vi "Rx_with scope_cal_TX.vi"() -> ()   [LabVIEW 2021]
uses:
  use with scope/states_for scope.ctl
  CTL/device_mode.ctl
  <instrlib>/niScope/Controls/niScope trigger source digital.ctl
  use with scope/scope trig type.ctl
  CTL/user config.ctl
  <vilib>/userdefined/High Color/nirio_resource_hc.ctl
  classes/5785_3.2GHz_one channel/5785_3.2GHz_one channel.lvclass
  C:/Users/PXIe8108_Demo/Documents/CHAIM DATA/chaim/5785_sync_for_elbit/tx_pulse/pulse Tx Folder_lv_21/EMEA_ADG_EW_Multi_Emitter_Scenarios/classes/device_type/device_type.lvclass
  classes/5785_2_x_1600MHz/5785_2_x_1600MHz.lvclass
  <instrlib>/niScope/Configure/Trigger/niScope Configure Trigger Edge.vi
  <instrlib>/niScope/Configure/Trigger/niScope Configure Trigger Digital.vi
  <instrlib>/niScope/Acquire/Fetch/niScope Multi Fetch WDT.vi
  <vilib>/Analysis/1siggen.llb/Ramp Pattern by Delta.vi
  classes/device_type/device_type.lvclass
  <vilib>/Analysis/NI_AALBase.lvlib
panel:
  out "delta distance":cluster{dbl[], dbl[]}[](graph)
  out "delta phase (deg)":cluster{dbl[], dbl[]}[](graph)
  in  "niqiest band":dbl[](array[numeric])=[0.0, 0.0, 0.0, 0.0, 0.0, 0.0, 0.0, 0.0, 0.0, 0.0, 0.0, 0.0, 0.0, 0.0, 0.0, 0.0, 0.0, 0.0]
  in  "clear":bool=TRUE
  out "saturate":bool
  out "delta phase(deg) 2":cluster{dbl[], dbl[]}[](graph)
  out "delta amp (dB) 2":cluster{dbl[], dbl[]}[](graph)
  in  "atenuattion (dB)":dbl format="%#_13g"
  in  "Min. Sample Rate":dbl=1250000000.0 format="%#.3p"
  in  "maximum input frequency":dbl=800000000.0 format="%#_13p"
  in  "input impedance":u32(ring)=2 items=["1 mega ohm"=0, "50 ohms"=2]
  in  "keep data":bool=TRUE
  in  "test mode":bool
  in  "save file":bool=TRUE
  in  "file path":path=path "C:/Users/PXIe8108_Demo/Documents/CHAIM DATA/chaim/5785_sync_for_elbit/tx_pulse/pulse Tx Folder_lv_21/EMEA_ADG_EW_Multi_Emitter_Scenarios/data/scope_cal_file.tdms"
  in  "num of recordes":dbl=18.0 format="%#_13g"
  in  "device type":T1=enum."5785 2*1.6GHz"
  in  "num of devices":dbl=2.0 format="%#_13g"
  in  "gen PDW file":bool
  in  "frequncy comb":cluster{"start":dbl, "end":dbl, "delta":dbl}={"start"=20000000.0, "end"=300000000.0, "delta"=1000000.0} {"delta" format="%#_6p"; "end" format="%#_6p"; "start" format="%#_6p"}
  in  "scope cal file":path=path "C:/Users/PXIe8108_Demo/Documents/CHAIM DATA/chaim/5785_sync_for_elbit/tx_pulse/pulse Tx Folder_lv_21/EMEA_ADG_EW_Multi_Emitter_Scenarios/data/scope_cal_file_5171_1234567.tdms"
  out "spectrum":cluster{"f0":dbl, "df":dbl, "magnitude":dbl[]}[](graph)=[{"f0"=0.0, "df"=10000.0, "magnitude"=array[62500 elements]}, {"f0"=0.0, "df"=10000.0, "magnitude"=array[62500 elements]}, {"f0"=0.0, "df"=10000.0, "magnitude"=array[62500 elements]}, {"f0"=0.0, "df"=10000.0, "magnitude"=array[62500 elements]}]
  in  "reset data":bool
  in  "loop mode":bool=TRUE
  out "state":T2=enum."run mesearment"
  in  "cal":bool
  in  "connection table (skip channel 0)":i32[](array[numeric])=[1, 2, 3, 4, 5, 6]
  out "delta amp (dB)":cluster{dbl[], dbl[]}[](graph)
  in  "Channel Name":string="0,1,2,3"
  in  "Resource Name":refnum<k15>="PXI1Slot6" caption="Resource Name(s)"
  in  "amplitude (dB)":dbl=-30.0 format="%#_13g"
  in  "record duration (s)":dbl=0.0001 format="%#_13p"
  out "scope":waveform(dbl)[](graph)=[{"t0"=timestamp(3784724283.659386 s since 1904-01-01), "dt"=8e-10, "Y"=array[125000 elements]}, {"t0"=timestamp(3784724283.659386 s since 1904-01-01), "dt"=8e-10, "Y"=array[125000 elements]}, {"t0"=timestamp(3784724283.659386 s since 1904-01-01), "dt"=8e-10, "Y"=array[125000 elements]}, {"t0"=timestamp(3784724283.659386 s since 1904-01-01), "dt"=8e-10, "Y"=array[125000 elements]}]
  # "scope delta detection"
  # "RF setup"
  # "HW setup"
  # "Rx Data"
  # "scope mapping:\nchannel 0 => 5785_02 _0 \nchannel 1 => 5785_01 _0 \nchannel 2 => 5785_01 _1 \nchannel 3 => 5785_00 _1"
  # "SW setup"
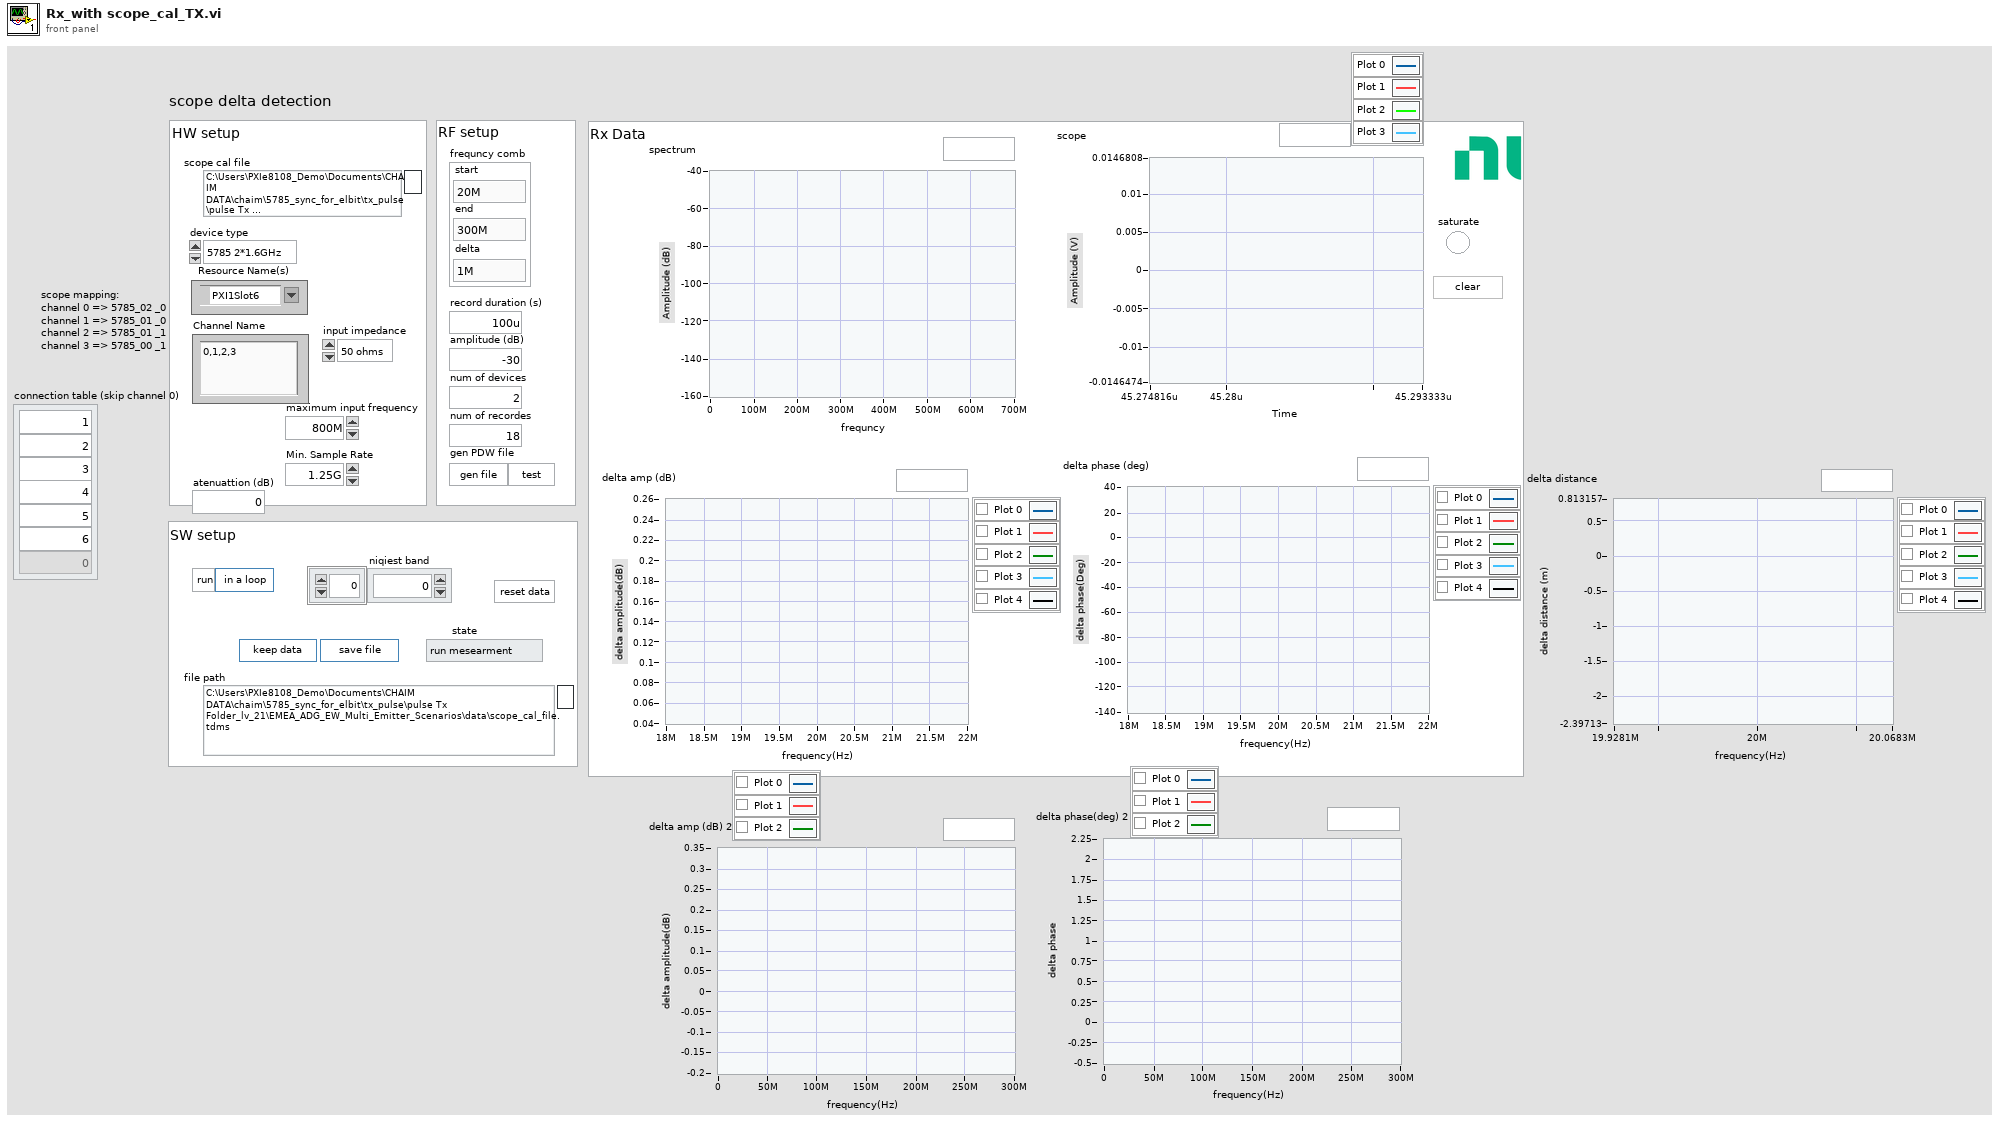
[diagram p1: front panel]
types:
  T1 = typedef "device_mode.ctl" = enum16{"5785 - 3.2GHz", "5785 2*1.6GHz", "P2P - VST", "USRP - 180MHz", "P2P Tx and Rx"}
  T2 = typedef "states_for scope.ctl" = enum16{"wait", "update ME config", "gen secenario", "INI ME", "INI scope", "trig", "close ME", "run mesearment", "save cal data", "get file data", "gen PDW file", "keep the data", "reset memory data", "prime the fifo"}
  T3 = typedef "niScope trigger source digital.ctl" = string
  T4 = typedef "scope trig type.ctl" = enum16{"digital", "analog"}
  T5 = cluster{"freqency":dbl[], "phase":dbl[], "amp":dbl[]}
  T6 = enum16{"open", "open or create", "create or replace", "create", "open (read-only)"}
  T7 = typedef "nirio_resource_hc.ctl" = tag
  T8 = typedef "user config.ctl" = cluster{"vst_device":refnum<k15>[], "RF gain ":dbl, "buffer size":u32, "center frequency (Hz) ":dbl, "P2P sample rate":dbl, "mode":enum16{"USRP - 180MHz", "5785 - 2*180MHz", "5785 - 3.2GHz", "P2P - VST"}, "devicess":T7[], "gen for df":bool, "Rx settings":cluster{"min PW         ":dbl, "max gap        ":dbl, "detection bar":dbl, "peak detect                        ":bool}, "use arb files":bool}
  T9 = cluster{"freqency":dbl[], "phase":dbl[], "amp":dbl[]}[]
  T10 = cluster{"frequncy":dbl, "d amp":dbl, "d phase":dbl}[]
  T11 = cluster{"frequncy":dbl, "d amp":dbl, "d phase":dbl}[][]
  T12 = typedef "PDW_lv2.ctl" = cluster{"t start":dbl, "frequency (Hz)":dbl, "duration (sec)":dbl, "mod type":T13, "mod depth":dbl, "trig":bool, "amp (lin)":dbl, "diraction (deg)":dbl, "phase(deg)":dbl}
  T13 = typedef "mode_type.ctl" = enum8{"CW", "from memory 1", "NC - cw", "LFM", "BPSK", "QPSK"}
  T14 = cluster{"Array":dbl[], "Array":dbl[], "Array":dbl[]}
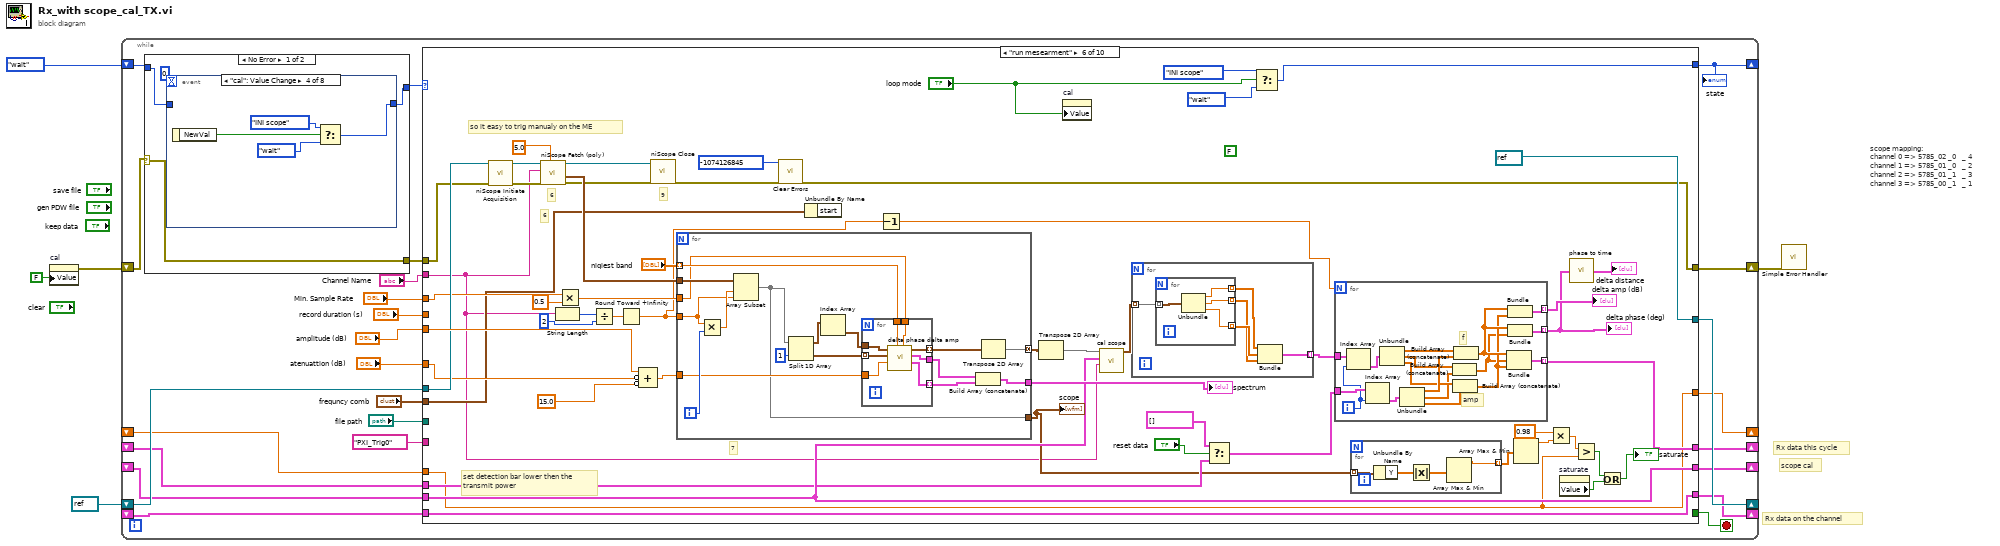
[diagram p0: block diagram]
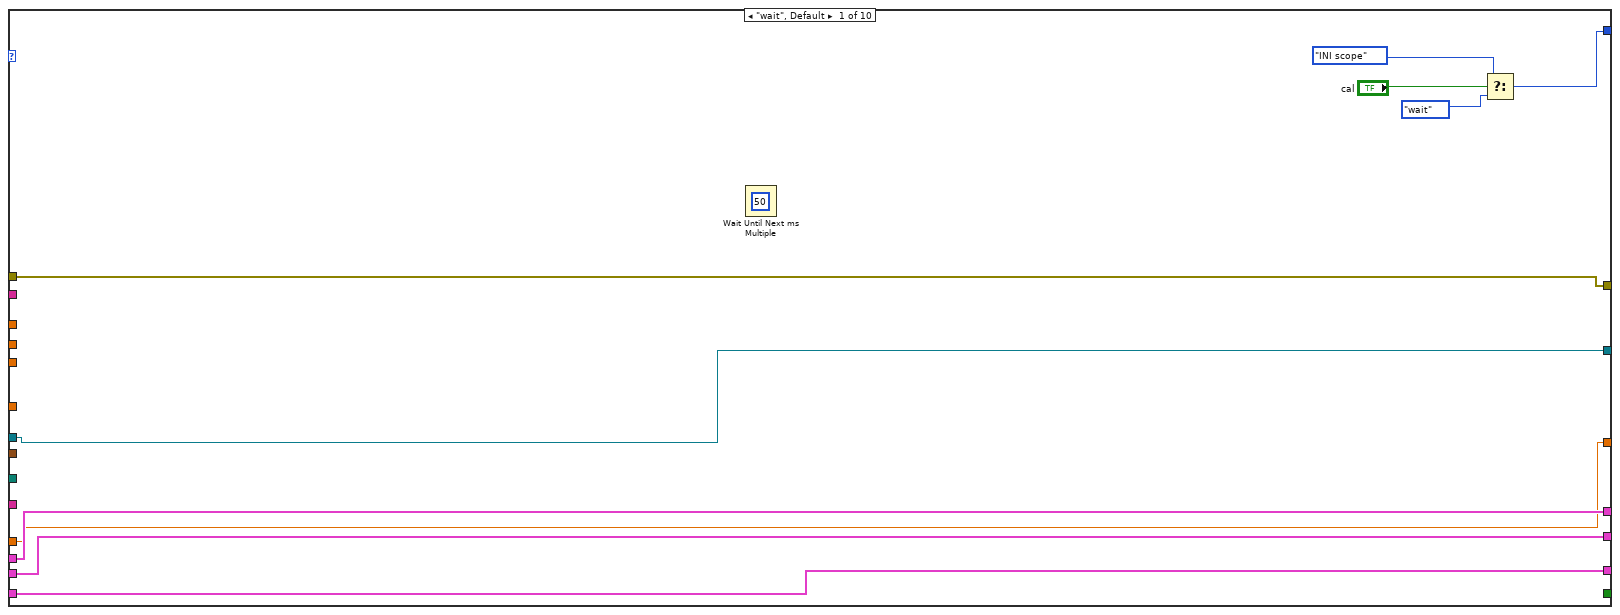
[diagram p2: hidden frame]
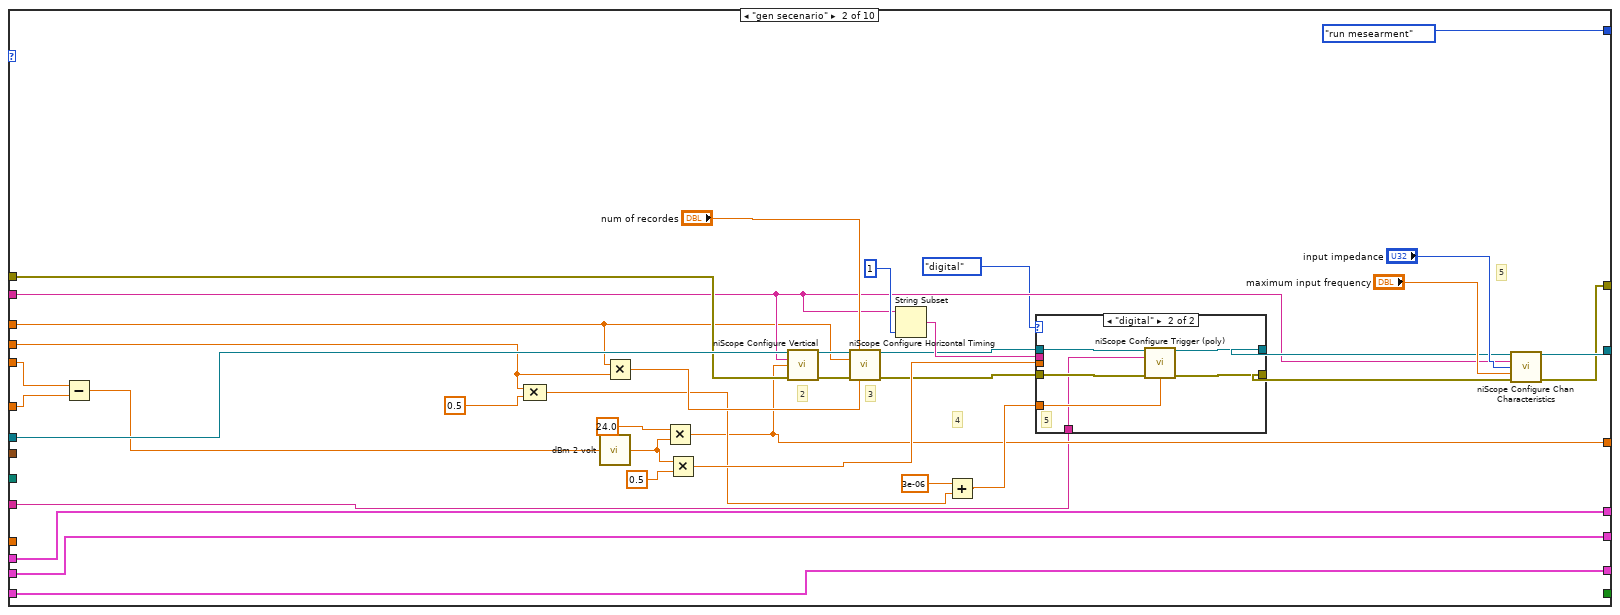
[diagram p3: hidden frame]
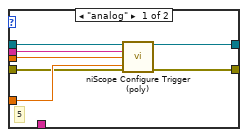
[diagram p4: hidden frame]
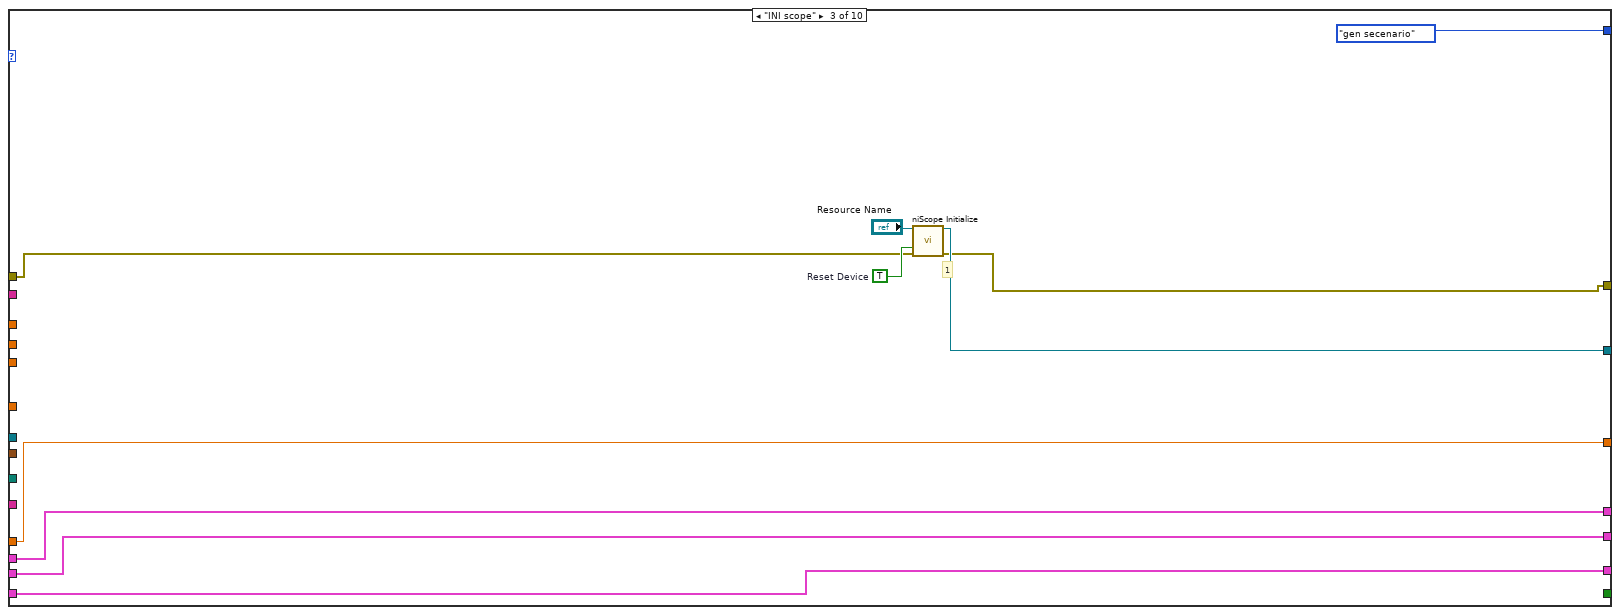
[diagram p5: hidden frame]
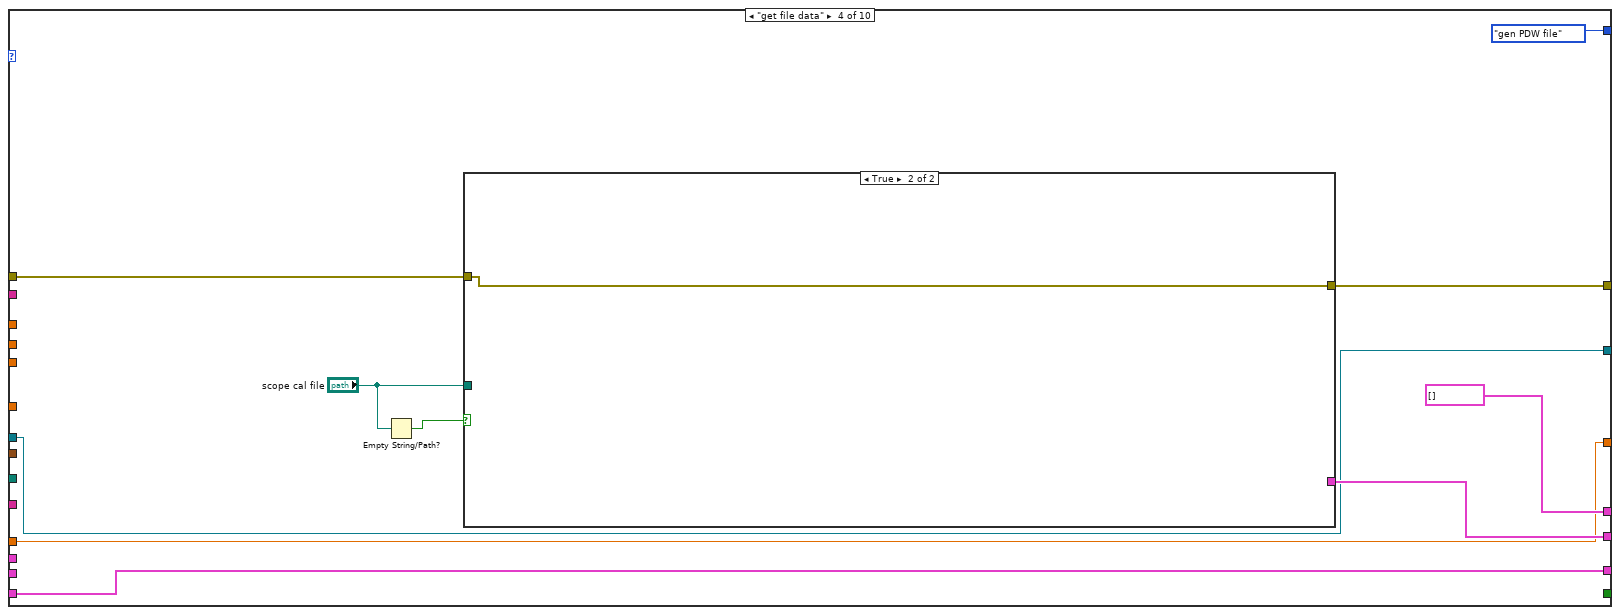
[diagram p6: hidden frame]
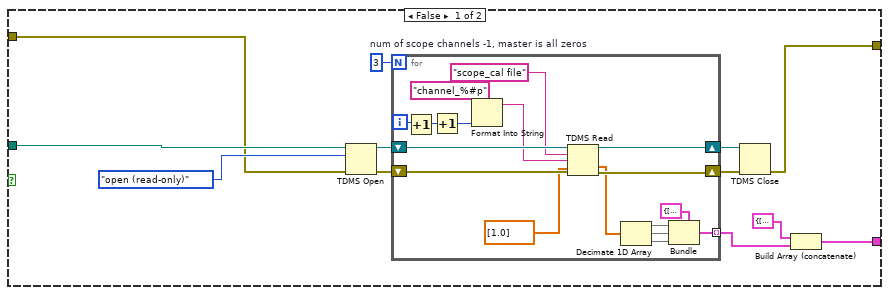
[diagram p7: hidden frame]
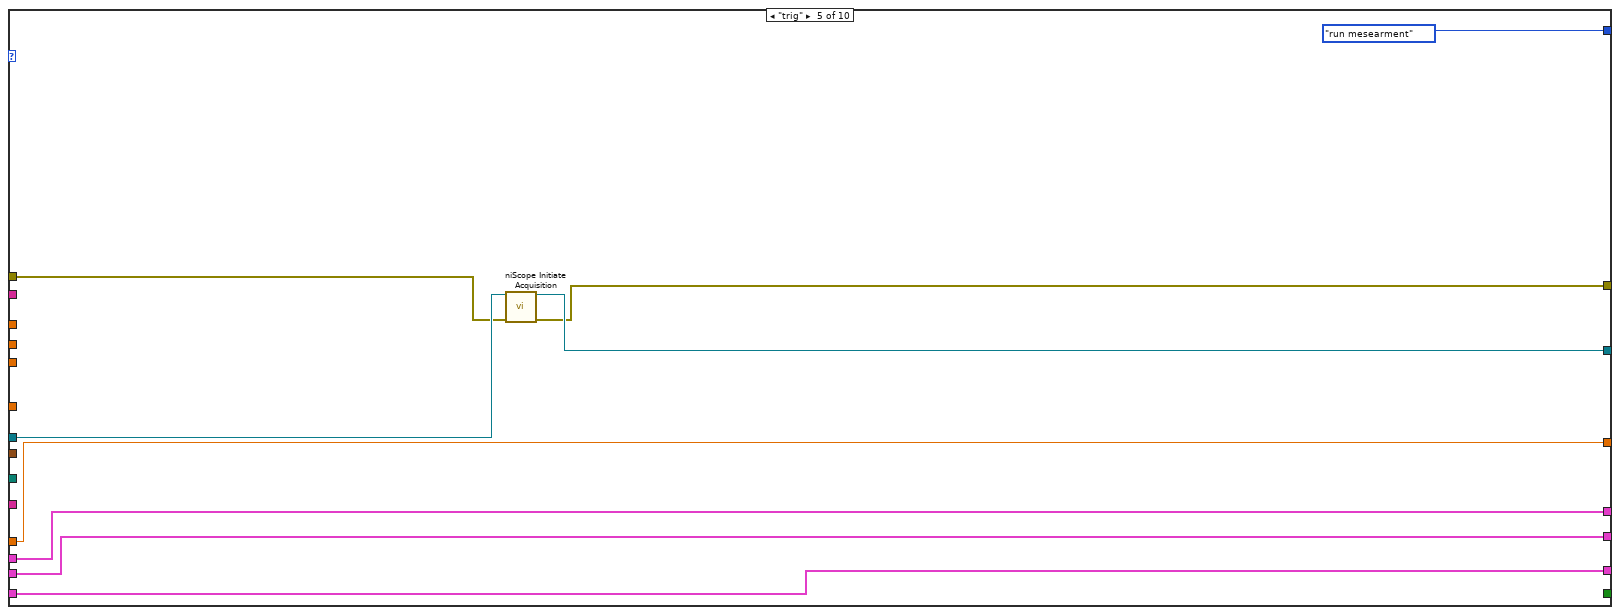
[diagram p8: hidden frame]
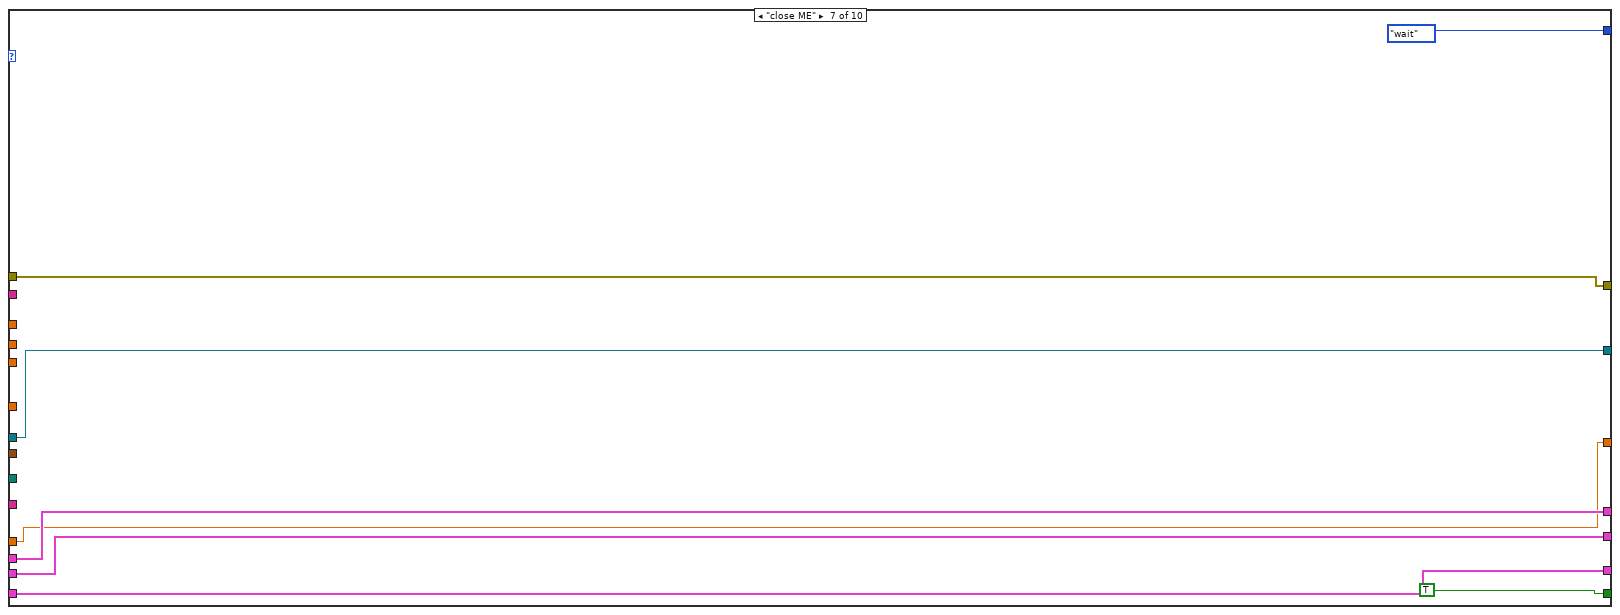
[diagram p9: hidden frame]
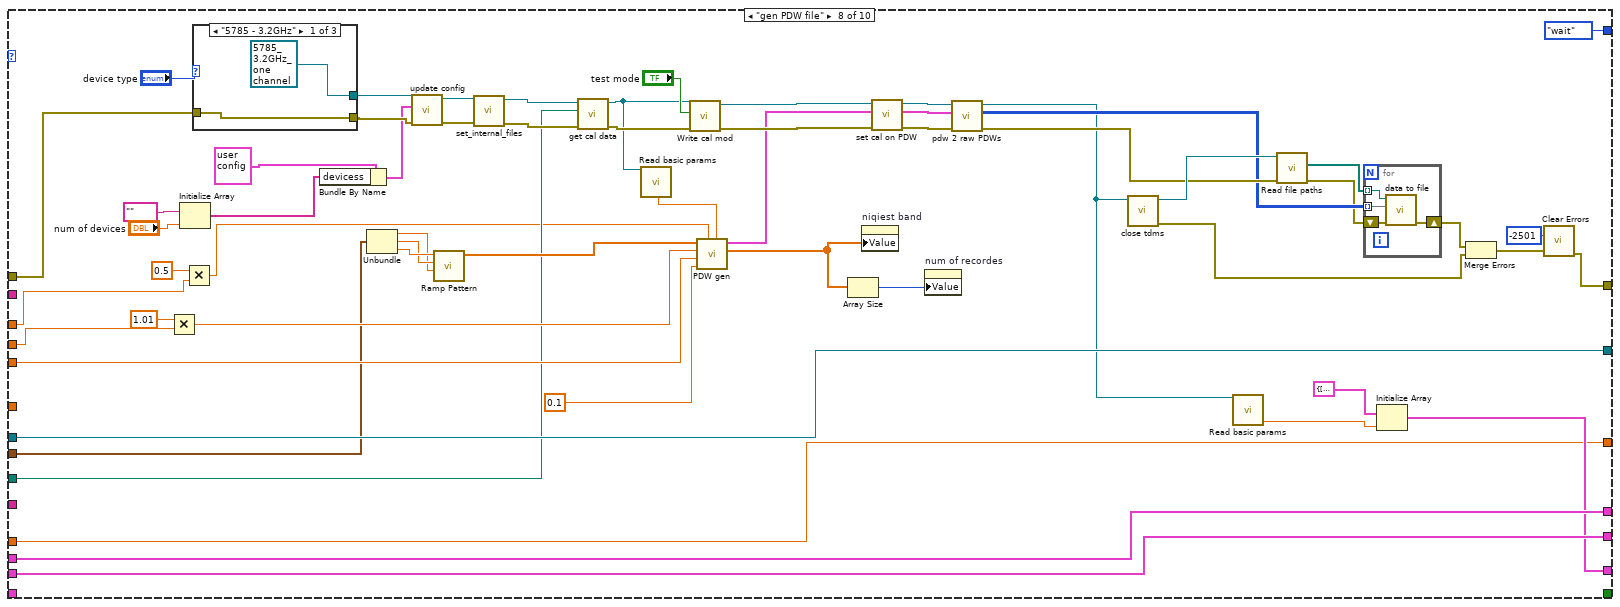
[diagram p10: hidden frame]
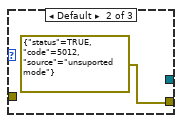
[diagram p11: hidden frame]
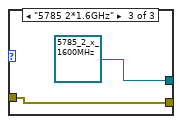
[diagram p12: hidden frame]
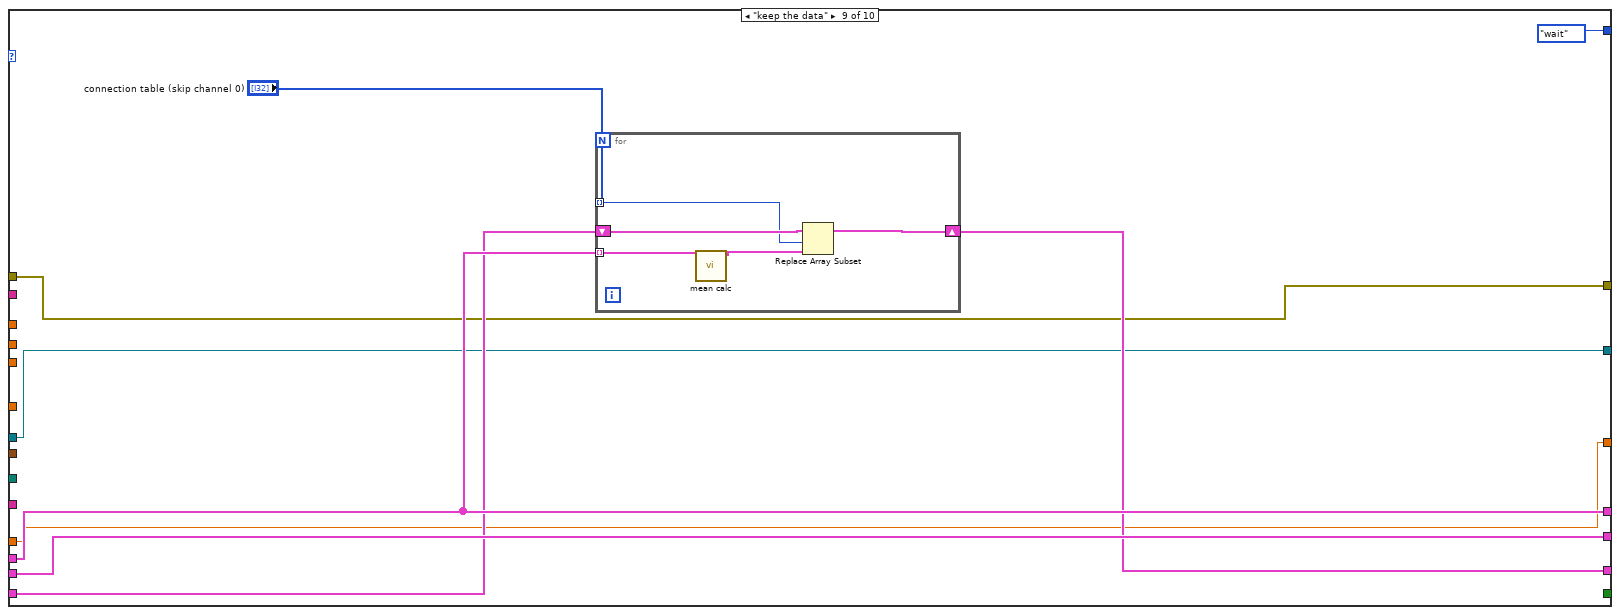
[diagram p13: hidden frame]
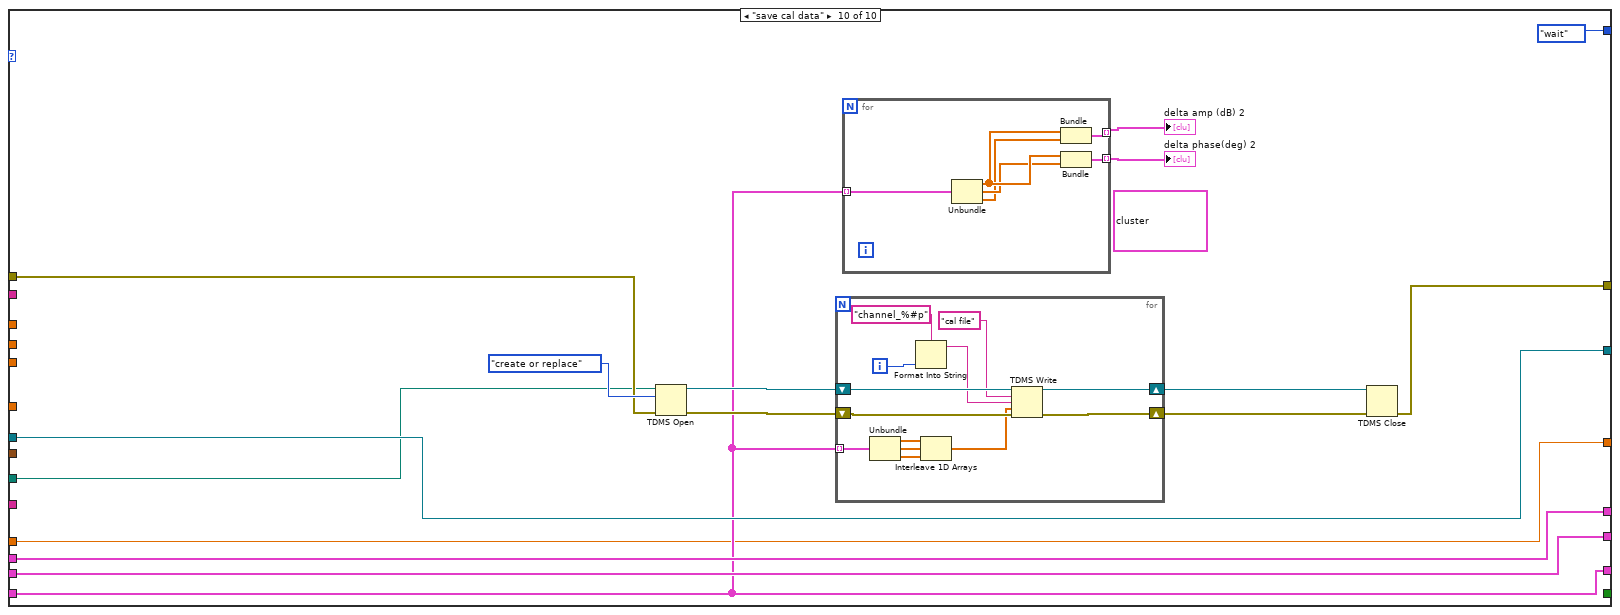
[diagram p14: hidden frame]
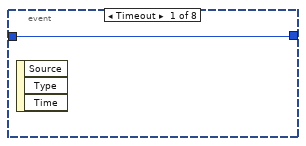
[diagram p15: hidden frame]
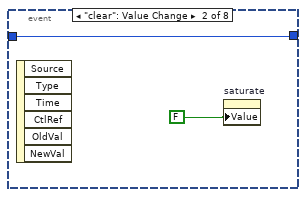
[diagram p16: hidden frame]
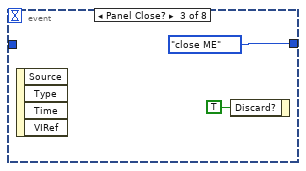
[diagram p17: hidden frame]
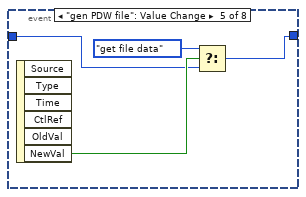
[diagram p18: hidden frame]
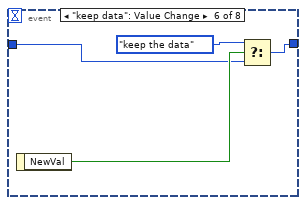
[diagram p19: hidden frame]
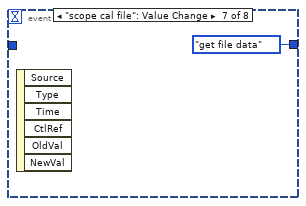
[diagram p20: hidden frame]
diagram:
  # "Rx data on the channel"
  # "Rx data this cycle"
  # "scope cal"
  # "scope mapping:\nchannel 0 => 5785_02 _0   _ 4\nchannel 1 => 5785_01 _0   _ 2 \nchannel 2 => 5785_01 _1   _ 3\nchannel 3 => 5785_00 _1   _ 1"
  n1 = property on="cal" class="Bool (strict)"("Value"=FALSE ("cal")) -> (error out=w1:errorcluster)  [unwired: 2 in, 1 out]
  n2 = while {
    shift-right: [w20] -> _
    shift-left: states_for_scope."wait" -> [w28]
    shift-right: [w26] -> w3
    shift-left: w1 -> [w30]
    shift-right: [w23] -> _
    shift-left: refnum<k15> refnum ("instrument handle out") -> [w22]
    shift-right: [w18] -> _
    shift-left: _ -> [w17]
    shift-right: [w16] -> _
    shift-left: _ -> [w15]
    shift-right: [w14] -> _
    shift-left: _ -> [w13]
    shift-right: [w10] -> _
    shift-left: _ -> [w9]
    stop <- w19 stop-if-true
    n3 = case shown="No Error" w30 {
      selector: w30 -> [w388 w410]
      tunnel: [w386 states_for_scope."close ME"] -> w29
      tunnel: w28 -> [w387 _]
      tunnel: [w388 errorcluster {"status"=FALSE, "code"=0, "source"=""} ("error IO")] -> w27
      frame No Error {
        n4 = event shown="[3] \"cal\": Value Change" {
          selector: _ -> [_ _ _ _ _ _ _ _]
          dyn-events: _ -> [_ _ _ _ _ _ _ _]
          timeout: 0 -> [_ _ _ _ _ _ _ _]
          tunnel: w387 -> [w389 w391 _ _ w400 w403 _ _]
          tunnel: [w389 w391 states_for_scope."close ME" w395 w399 w402 states_for_scope."get file data" ("f") states_for_scope."save cal data" ("f")] -> w386
          event Timeout {
            n5 = event-data() -> ()  [unwired: 1 in, 3 out]
          }
          event "clear": Value Change {
            n6 = event-data() -> ()  [unwired: 1 in, 6 out]
            n7 = property on="saturate" class="Bool (strict)"("Value"=FALSE ("clear")) -> ()  [unwired: 2 in, 2 out]
          }
          event Panel Close? {
            n8 = event-data() -> ()  [unwired: 1 in, 4 out]
            n9 = event-data("Discard?"=TRUE) -> ()  [unwired: 1 in, 1 out]
          }
          event "cal": Value Change {
            n10 = event-data() -> ("NewVal"=w397:bool)  [unwired: 1 in]
            n11 = Select(t=states_for_scope."INI scope", s=w397, f=states_for_scope."wait") -> (s? t:f=w395:T2)
          }
          event "gen PDW file": Value Change {
            n12 = event-data() -> ("NewVal"=w401:bool)  [unwired: 1 in, 5 out]
            n13 = Select(t=states_for_scope."get file data", s=w401, f=w400) -> (s? t:f=w399:T2)
          }
          event "keep data": Value Change {
            n14 = event-data() -> ("NewVal"=w405:bool)  [unwired: 1 in]
            n15 = Select(t=states_for_scope."keep the data" ("f"), s=w405, f=w403) -> (s? t:f=w402:T2)
          }
          event "scope cal file": Value Change {
            n16 = event-data() -> ()  [unwired: 1 in, 6 out]
          }
          event "save file": Value Change {
            n17 = event-data() -> ()  [unwired: 1 in, 6 out]
          }
        }
      }
      frame Error {
        n18 = call <vilib>:"Simple Error Handler.vi"("error in (no error)"=w410) -> ()  [unwired: 4 in, 5 out]
      }
    }
    n19 = case shown="\"run mesearment\"" w29 {
      tunnel: w27 -> [w40 w63 w96 w108 w147 w194 w265 w311 w337 w360]
      tunnel: [w40 w56 w98 w109 w148 w190 w265 w316 w337 w359] -> w26
      tunnel: "record duration (s)" -> [_ w67 _ _ _ _ _ w305 _ _]
      tunnel: "amplitude (dB)" -> [_ w47 _ _ _ w197 _ w302 _ _]
      tunnel: [w39 w57 w99 w110 w149 refnum<k15> refnum ("instrument handle out") w266 w300 w338 w357] -> w23
      tunnel: w22 -> [w39 w68 _ w110 w150 w196 w266 w300 w338 w357]
      tunnel: "Channel Name" -> [_ w53 _ _ _ w158 _ _ _ _]
      tunnel: [w32 states_for_scope."run mesearment" states_for_scope."gen secenario" states_for_scope."gen PDW file" states_for_scope."run mesearment" w198 states_for_scope."wait" states_for_scope."wait" states_for_scope."wait" states_for_scope."wait"] -> w20
      tunnel: [_ _ _ _ _ _ TRUE _ _ _] -> w19
      tunnel: [w38 w62 w95 w111 w145 w179 w264 w298 w344 w355] -> w18
      tunnel: w17 -> [w38 w62 w95 _ w145 w179 w264 w298 w344 w355]
      tunnel: [w37 w61 w94 cluster{dbl[], dbl[], dbl[]}[] [] w144 w178 w263 w299 w341 w356] -> w16
      tunnel: w15 -> [w37 w61 w94 _ w144 w177 w263 w299 w341 w356]
      tunnel: [w36 w52 w93 w106 w143 w176 w262 w289 w339 w354] -> w14
      tunnel: w13 -> [w36 w52 w93 w106 w143 w176 w262 _ w340 w354]
      tunnel: "atenuattion (dB)" -> [_ w46 _ _ _ w174 _ _ _ _]
      tunnel: "file path" -> [_ _ _ _ _ _ _ w279 _ w351]
      tunnel: [w31 w44 w92 w104 w142 w170 w261 w278 w336 w350] -> w10
      tunnel: w9 -> [w31 _ w92 w104 w142 w170 w261 w278 w336 w350]
      tunnel: "Min. Sample Rate" -> [_ w43 _ _ _ w162 _ w276 _ _]
      tunnel: "frequncy comb" -> [_ _ _ _ _ w159 _ w272 _ _]
      tunnel: T3 "PXI_Trig0" ("trigger source") -> [_ w42 _ _ _ _ _ _ _ _]
      frame "wait", Default {
        n20 = Wait Until Next ms Multiple(millisecond multiple=u32 50) -> ()  [unwired: 1 out]
        n21 = Select(t=states_for_scope."INI scope", s="cal", f=states_for_scope."wait") -> (s? t:f=w32:T2)
      }
      frame "gen secenario" {
        # "5"
        # "4"
        # "3"
        # "2"
        n22 = Subtract(x=w47, y=w46) -> (x-y=w45:dbl)
        n23 = Compound Arithmetic op=MULTIPLY(w67, 0.5 ("value")) -> (w50:dbl)
        n24 = call "dBm 2 volt.vi"("dBm"=w45) -> ("V"=w76:dbl)
        n25 = Multiply(x=w43, y=w67) -> (x*y=w78:dbl)
        n26 = Multiply(x=24.0, y=w76) -> (x*y=w44:dbl)
        n27 = Multiply(x=w76, y=0.5) -> (x*y=w77:dbl)
        n28 = call <instrlib>:"niScope Configure Vertical.vi"("instrument handle"=w68, "channels"=w53, "vertical range"=w44, "error in"=w63) -> ("instrument handle out"=w65:refnum<k15>, "error out"=w64:errorcluster)  [unwired: 10 in]
        n29 = call <instrlib>:"niScope Configure Horizontal Timing.vi"("instrument handle"=w65, "number of records"="num of recordes", "min sample rate"=w43, "error in"=w64, "min record length"=w78) -> ("instrument handle out"=w74:refnum<k15>, "error out"=w73:errorcluster)  [unwired: 9 in]
        n30 = String Subset(string=w53, length (rest)=1 ("length (rest)")) -> (substring=w75:string)  [unwired: 1 in]
        n31 = Add(x=3e-06, y=w50) -> (x+y=w48:dbl)
        n32 = case shown="\"digital\"" scope_trig_type."digital" {
          tunnel: w77 -> [w85 _]
          tunnel: w48 -> [w84 w87]
          tunnel: w75 -> [w83 _]
          tunnel: w74 -> [w82 w91]
          tunnel: w73 -> [w81 w90]
          tunnel: [w80 w89] -> w58
          tunnel: [w79 w88] -> w55
          tunnel: w42 -> [_ w86]
          frame "analog" {
            # "5"
            n33 = call-poly <instrlib>:"niScope Configure Trigger (poly).vi"("instrument handle"=w82, "trigger source"=w83, "trigger level"=w85, "error in"=w81, "trigger delay"=w84) -> ("instrument handle out"=w80:refnum<k15>, "error out"=w79:errorcluster)  [unwired: 9 in]
          }
          frame "digital" {
            # "5"
            n34 = call-poly <instrlib>:"niScope Configure Trigger (poly).vi"("instrument handle"=w91, "trigger source"=w86, "error in"=w90, "trigger delay"=w87) -> ("instrument handle out"=w89:refnum<k15>, "error out"=w88:errorcluster)  [unwired: 10 in]
          }
        }
        n35 = call <instrlib>:"niScope Configure Chan Characteristics.vi"("instrument handle"=w58, "channels"=w53, "input impedance"="input impedance", "maximum input frequency"="maximum input frequency", "error in"=w55) -> ("instrument handle out"=w57:refnum<k15>, "error out"=w56:errorcluster)  [unwired: 9 in]
      }
      frame "INI scope" {
        w100 = TRUE  # Reset Device
        # "1"
        n36 = call <instrlib>:"niScope Initialize.vi"("resource name"="Resource Name", "reset device"=w100, "error in"=w96) -> ("instrument handle"=w99:refnum<k15>, "error out"=w98:errorcluster)  [unwired: 11 in]
      }
      frame "get file data" {
        n37 = Empty String/Path?(string/path="scope cal file") -> (empty?=w102:bool)
        n38 = case shown="True" w102 {
          tunnel: "scope cal file" -> [w118 _]
          tunnel: [w114 _] -> w111
          tunnel: [w113 w141] -> w109
          tunnel: w108 -> [w112 w141]
          frame False {
            w116 = 3  # num of scope channels -1, master is all zeros
            n39 = TDMS Open(8:w112, 10:T6."open (read-only)" ("operation (0:open)"), 11:w118) -> (0:w121:errorcluster, 3:w120:refnum<k34>)  [unwired: 4 in]
            n40 = for {
              N: w116 -> [_]
              shift-right: [w138] -> w122
              shift-left: w120 -> [w140]
              shift-right: [w137] -> w123
              shift-left: w121 -> [w139]
              tunnel: [w127] -> w119 mode=indexing
              i -> [w126]
              n41 = Increment(x=w126) -> (x+1=w124:i32)
              n42 = Increment(x=w124) -> (x+1=w125:i32)
              n43 = Format Into String(format string="channel_%#p", w125) -> (resulting string=w135:string)  [unwired: 2 in, 1 out]
              n44 = TDMS Read(0:w140, 5:"scope_cal file" ("group name in (Untitled)"), 7:w135, 11:w139, 12:dbl[] [1.0] ("interleaved array")) -> (4:w138:refnum<k34>, 10:w132:dbl[], 15:w137:errorcluster)  [unwired: 3 in, 3 out]
              n45 = Decimate 1D Array(w132) -> (w130:dbl[], w129:dbl[], w128:dbl[])
              n46 = Bundle(cluster=T5 {"freqency"=[], "phase"=[], "amp"=[]}, "freqency"=w130, "phase"=w129, "amp"=w128) -> (w127:T5)
            }
            n47 = TDMS Close(8:w123, 11:w122) -> (0:w113:errorcluster)  [unwired: 1 out]
            n48 = Build Array (concatenate)(T5 {"freqency"=[], "phase"=[], "amp"=[]}, w119) -> (w114:T9)
          }
          frame True {
          }
        }
      }
      frame "trig" {
        n49 = call <instrlib>:"niScope Initiate Acquisition.vi"("instrument handle"=w150, "error in"=w147) -> ("instrument handle out"=w149:refnum<k15>, "error out"=w148:errorcluster)  [unwired: 12 in]
      }
      frame "run mesearment" {
        (unwired) FALSE ("cal mode")
        # "so it easy to trig manualy on the ME"
        # "set detection bar lower then the\ntransmit power"
        # "6"
        # "9"
        # "7"
        # "6"
        n50 = call <instrlib>:"niScope Initiate Acquisition.vi"("instrument handle"=w196, "error in"=w194) -> ("instrument handle out"=w195:refnum<k15>, "error out"=w193:errorcluster)  [unwired: 12 in]
        n51 = call-poly <instrlib>:"niScope Fetch (poly).vi"("timeout"=5.0, "error in"=w193, "channels"=w158, "instrument handle"=w195) -> ("error out"=w202:errorcluster, "wfm"=w204:waveform(dbl)[], "instrument handle out"=w201:refnum<k15>)  [unwired: 4 in, 1 out]
        n52 = String Length(string=w158) -> (length=w156:i32)
        n53 = Multiply(x=w162, y=0.5) -> (x*y=w160:dbl)
        n54 = Divide(x=w156, y=2 ("x")) -> (x/y=w157:dbl)
        n55 = Round Toward +Infinity(x=w157) -> (ceil(x): smallest int >= x=w154:dbl)
        n56 = Compound Arithmetic op=ADD(w197, invert w174, invert 15.0 ("value")) -> (w203:dbl)
        n57 = call <instrlib>:"niScope Close.vi"("instrument handle"=w201, "error in"=w202) -> ("error out"=w191:errorcluster)  [unwired: 13 in]
        n58 = for {
          tunnel: w204 -> [w243]
          tunnel: w203 -> [w237]
          tunnel: [w235] -> w205 mode=concatenating
          tunnel: [w234] -> w172
          tunnel: [w231] -> w182
          tunnel: "niqiest band" -> [w230] mode=indexing
          tunnel: w160 -> [w229]
          tunnel: w154 -> [w228]
          i -> [w242]
          n59 = Multiply(x=w228, y=w242) -> (x*y=w241:dbl)
          n60 = Array Subset(array=w243, index=w241, length=w228) -> (w234:waveform(dbl)[])
          n61 = Split 1D Array(array=w234, index=1) -> (first subarray=w227:waveform(dbl)[], second subarray=w238:waveform(dbl)[])
          n62 = Index Array(array=w227) -> (element=w239:waveform(dbl))  [unwired: 1 in]
          n63 = for {
            tunnel: w239 -> [w251]
            tunnel: w238 -> [w250] mode=indexing
            tunnel: w237 -> [w249]
            tunnel: [w248] -> w236 mode=indexing
            tunnel: [w247] -> w233
            tunnel: [w246] -> w232 mode=indexing
            tunnel: w230 -> [w245]
            tunnel: w229 -> [w244]
            n64 = call "delta phase delta amp.vi"("niqiest frequecy"=w244, "niqiest band"=w245, "detection bar"=w249, "signal in 2"=w250, "signal in 1"=w251) -> ("PSD 1"=w246:cluster{"f0":dbl, "df":dbl, "magnitude":dbl[]}, "PSD 0"=w247:cluster{"f0":dbl, "df":dbl, "magnitude":dbl[]}, "cal data"=w248:T10)  [unwired: 4 in]
          }
          n65 = Build Array (concatenate)(w233, w232) -> (w231:cluster{"f0":dbl, "df":dbl, "magnitude":dbl[]}[])
          n66 = Transpose 2D Array(2D array=w236) -> (transposed array=w235:T11)
        }
        "scope" <- w172
        "spectrum" <- w182
        n67 = call <vilib>:"Clear Errors.vi"("error in (no error)"=w191, "specific error code to clear (0: all)"=-1074126845) -> ("error out"=w190:errorcluster)  [unwired: 4 in, 1 out]
        n68 = Unbundle By Name(w159) -> ()  [unwired: 1 out]
        n69 = Decrement(x=w154) -> (x-1=w153:dbl)
        n70 = Transpose 2D Array(2D array=w205) -> (transposed array=w181:T11)
        n71 = property on="cal" class="Bool (strict)"("Value"="loop mode") -> ()  [unwired: 2 in, 2 out]
        n72 = call "cal scope.vi"("Channel Name"=w158, "scope cal data"=w179, "measured data"=w181) -> ("measured and cal data"=w180:T11)  [unwired: 8 in]
        n73 = for {
          tunnel: w180 -> [w256] mode=indexing
          tunnel: [w252] -> w187 mode=indexing
          n74 = for {
            tunnel: w256 -> [w260] mode=indexing
            tunnel: [w259] -> w255 mode=indexing
            tunnel: [w258] -> w254 mode=indexing
            tunnel: [w257] -> w253 mode=indexing
            n75 = Unbundle(w260) -> ("frequncy"=w259:dbl, "d amp"=w257:dbl, "d phase"=w258:dbl)
          }
          n76 = Bundle(w255, w254, w253) -> (w252:cluster{dbl[], dbl[], dbl[]})  [unwired: 1 in]
        }
        n77 = Select(t=cluster{dbl[], dbl[], dbl[]}[] [], s="reset data", f=w177) -> (s? t:f=w184:cluster{dbl[], dbl[], dbl[]}[])
        n78 = Select(t=states_for_scope."INI scope", s="loop mode", f=states_for_scope."wait") -> (s? t:f=w198:T2)
        n79 = for {
          N: w153 -> [_]
          tunnel: w187 -> [w211]
          tunnel: w184 -> [w226]
          tunnel: [w218] -> w178 mode=indexing
          tunnel: [w217] -> w186 mode=indexing
          tunnel: [w216] -> w152 mode=indexing
          i -> [w210]
          # "amp"
          # "f"
          n80 = Index Array(array=w211, index=w210) -> (element=w212:cluster{dbl[], dbl[], dbl[]})
          n81 = Index Array(array=w226, index=w210) -> (element=w225:cluster{dbl[], dbl[], dbl[]})
          n82 = Unbundle(w212) -> (w224:dbl[], w222:dbl[], w221:dbl[])
          n83 = Unbundle(w225) -> (w223:dbl[], w220:dbl[], w219:dbl[])
          n84 = Build Array (concatenate)(w222, w220) -> (w213:dbl[])
          n85 = Build Array (concatenate)(w221, w219) -> (w214:dbl[])
          n86 = Build Array (concatenate)(w224, w223) -> (w215:dbl[])
          n87 = Bundle(w215, w213, w214) -> (w218:cluster{dbl[], dbl[], dbl[]})  [unwired: 1 in]
          n88 = Bundle(w215, w214) -> (w217:cluster{dbl[], dbl[]})  [unwired: 1 in]
          n89 = Bundle(w215, w213) -> (w216:cluster{dbl[], dbl[]})  [unwired: 1 in]
        }
        "delta amp (dB)" <- w186
        "delta phase (deg)" <- w152
        n90 = for {
          tunnel: w172 -> [w209] mode=indexing
          tunnel: [w208] -> w171 mode=indexing
          n91 = Unbundle By Name(w209) -> ("Y"=w207:dbl[])
          n92 = Absolute Value(x=w207) -> (abs(x)=w206:dbl[])
          n93 = Array Max & Min(array=w206) -> (max value=w208:dbl)  [unwired: 3 out]
        }
        n94 = Array Max & Min(array=w171) -> (max value=w169:dbl)  [unwired: 3 out]
        n95 = Multiply(x=0.98, y=w169) -> (x*y=w167:dbl)
        n96 = property on="saturate" class="Bool (strict)"() -> ("Value"=w166:bool)  [unwired: 2 in, 2 out]
        n97 = call "phase to time.vi"("data"=w152) -> ("data"=→"delta distance":cluster{"Array":dbl[], "Array":dbl[]}[])
        n98 = Greater?(x=w167, y=w170) -> (0:w165:bool)
        n99 = Or(x=w165, y=w166) -> (x .or. y?=→"saturate":bool)
      }
      frame "close ME" {
      }
      frame "gen PDW file" {
        n100 = Multiply(x=1.01, y=w305) -> (x*y=w303:dbl)
        n101 = Initialize Array(T7 "" ("resource name"), "num of devices") -> (w294:T7[])
        n102 = Multiply(x=0.5, y=w276) -> (x*y=w275:dbl)
        n103 = case shown="\"5785 - 3.2GHz\"" "device type" {
          tunnel: [refnum<class "5785_3.2GHz_one channel.lvclass"> refnum ("5785_3.2GHz_one channel.lvclass") _ refnum<class "5785_2_x_1600MHz.lvclass"> refnum ("5785_2_x_1600MHz.lvclass")] -> w312
          tunnel: w311 -> [w327 _ w330]
          tunnel: [w327 errorcluster {"status"=TRUE, "code"=5012, "source"="unsuported mode"} ("error IO") w330] -> w310
          frame "5785 - 3.2GHz" {
          }
          frame Default {
          }
          frame "5785 2*1.6GHz" {
          }
        }
        n104 = Bundle By Name(cluster=T8 {"vst_device"=["VST_1", "VST_2"], "RF gain "=10.0, "buffer size"=524288, "center frequency (Hz) "=1000000000.0, "P2P sample rate"=200000000.0, "mode"=enum."5785 - 2*180MHz", "devicess"=["IF_transiver_0", "IF_transiver_1", "IF_transiver_2"], "gen for df"=TRUE, "Rx settings"={"min PW         "=0.0, "max gap        "=0.0, "detection bar"=0.0, "peak detect                        "=FALSE}, "use arb files"=FALSE} ("user configurations"), "devicess"=w294) -> (w293:T8)
        n105 = Unbundle(w272) -> ("start"=w307:dbl, "end"=w308:dbl, "delta"=w309:dbl)
        n106 = call-dynamic "update config.vi"("error in (no error)"=w310, "user configurations"=w293, "device_type in"=w312) -> ("error out"=w314:errorcluster, "device_type out"=w315:refnum<class "device_type.lvclass">)  [unwired: 5 in, 2 out]
        n107 = call-poly <vilib>:"Ramp Pattern.vi"("start"=w307, "end"=w308, "delta"=w309) -> ("Ramp Pattern"=w306:dbl[])  [unwired: 6 in, 2 out]
        n108 = call-dynamic "set_internal_files.vi"("error in (no error)"=w314, "device_type in"=w315) -> ("error out"=w281:errorcluster, "device_type out"=w282:refnum<class "device_type.lvclass">)  [unwired: 8 in]
        n109 = call-dynamic "get cal data.vi"("error in (no error)"=w281, "cal file path"=w279, "device_type in"=w282) -> ("error out"=w280:errorcluster, "device_type out"=w270:refnum<class "device_type.lvclass">)  [unwired: 7 in]
        n110 = call-dynamic "Read basic params.vi"("device_type in"=w270) -> ("number of channels"=w269:dbl)  [unwired: 11 in, 7 out]
        n111 = call-dynamic "Write cal mod.vi"("error in (no error)"=w280, "apply cal data"="test mode", "device_type in"=w270) -> ("error out"=w286:errorcluster, "device_type out"=w287:refnum<class "device_type.lvclass">)  [unwired: 7 in]
        n112 = call "PDW gen.vi"("num of channels"=w269, "niqiest freqency"=w275, "D.C"=0.1, "pulse amplitude"=w302, "pulse duration"=w303, "frequency list"=w306) -> ("niqiest band"=w273:dbl[], "PDWs on channels"=w271:cluster{T12[]}[])  [unwired: 4 in]
        n113 = Array Size(array=w273) -> (size(s)=w274:i32)
        n114 = property on="niqiest band" class="Arr (strict)"("Value"=w273) -> ()  [unwired: 2 in, 2 out]
        n115 = call "set cal on PDW.vi"("error in (no error)"=w286, "PDWs on channels"=w271, "device_type in"=w287) -> ("error out"=w285:errorcluster, "PDWs on channels"=w284:cluster{T12[]}[], "device_type out"=w283:refnum<class "device_type.lvclass">)  [unwired: 6 in]
        n116 = property on="num of recordes" class="DigNum (strict)"("Value"=w274) -> ()  [unwired: 2 in, 2 out]
        n117 = call-dynamic "pdw 2 raw PDWs.vi"("error in (no error)"=w285, "PDWs on channels"=w284, "device_type in"=w283) -> ("error out"=w322:errorcluster, "Array"=w320:u64[][], "device_type out"=w290:refnum<class "device_type.lvclass">)  [unwired: 6 in]
        n118 = call-dynamic "close tdms.vi"("device_type in"=w290) -> ("error out"=w325:errorcluster, "device_type out"=w323:refnum<class "device_type.lvclass">)  [unwired: 9 in]
        n119 = call-dynamic "Read basic params.vi"("device_type in"=w290) -> ("number of channels"=w291:dbl)  [unwired: 11 in, 7 out]
        n120 = call-dynamic "Read file paths.vi"("error in (no error)"=w322, "device_type in"=w323) -> ("error out"=w319:errorcluster, "file paths"=w321:path[])  [unwired: 6 in, 2 out]
        n121 = for {
          tunnel: w320 -> [w333] mode=indexing
          shift-right: [w334] -> w324
          shift-left: w319 -> [w335]
          tunnel: w321 -> [w332] mode=indexing
          n122 = call "data to file.vi"("error in (no error)"=w335, "Array"=w333, "Path"=w332) -> ("error out"=w334:errorcluster)  [unwired: 8 in]
        }
        n123 = Initialize Array(cluster{dbl[], dbl[], dbl[]} {[], [], []}, w291) -> (w289:cluster{dbl[], dbl[], dbl[]}[])
        n124 = Merge Errors(w324, w325) -> (w326:errorcluster)
        n125 = call <vilib>:"Clear Errors.vi"("error in (no error)"=w326, "specific error code to clear (0: all)"=-2501) -> ("error out"=w316:errorcluster)  [unwired: 4 in, 1 out]
      }
      frame "keep the data" {
        n126 = for {
          tunnel: "connection table (skip channel 0)" -> [w348] mode=indexing
          tunnel: w341 -> [w346] mode=indexing
          shift-right: [w347] -> w339
          shift-left: w340 -> [w349]
          n127 = call "mean calc.vi"("Cluster in"=w346) -> ("Cluster out"=w345:T14)  [unwired: 10 in]
          n128 = Replace Array Subset(array=w349, new element=w345, index=w348) -> (w347:cluster{dbl[], dbl[], dbl[]}[])
        }
      }
      frame "save cal data" {
        (unwired) cluster{dbl[], dbl[]}[] [{[], []}, {array[562 elements], array[562 elements]}, {array[562 elements], array[562 elements]}, {array[562 elements], array[562 elements]}, {[], []}, {[], []}] ("delta amp (dB) 2")
        n129 = TDMS Open(8:w360, 10:T6."create or replace" ("operation (0:open)"), 11:w351) -> (0:w364:errorcluster, 3:w365:refnum<k34>)  [unwired: 4 in]
        n130 = for {
          shift-right: [w382] -> w363
          shift-left: w365 -> [w384]
          shift-right: [w381] -> w362
          shift-left: w364 -> [w383]
          tunnel: w354 -> [w375] mode=indexing
          i -> [w379]
          n131 = Unbundle(w375) -> (w374:dbl[], w373:dbl[], w372:dbl[])
          n132 = Format Into String(format string="channel_%#p", w379) -> (resulting string=w377:string)  [unwired: 2 in, 1 out]
          n133 = Interleave 1D Arrays(w374, w373, w372) -> (w380:dbl[])
          n134 = TDMS Write(0:w384, 5:"cal file" ("group name in (Untitled)"), 7:w377, 9:w380, 11:w383) -> (4:w382:refnum<k34>, 15:w381:errorcluster)  [unwired: 1 in, 2 out]
        }
        n135 = for {
          tunnel: w354 -> [w366] mode=indexing
          tunnel: [w368] -> w353 mode=indexing
          tunnel: [w367] -> w352 mode=indexing
          n136 = Unbundle(w366) -> (w371:dbl[], w370:dbl[], w369:dbl[])
          n137 = Bundle(w371, w369) -> (w368:cluster{dbl[], dbl[]})  [unwired: 1 in]
          n138 = Bundle(w371, w370) -> (w367:cluster{dbl[], dbl[]})  [unwired: 1 in]
        }
        "delta amp (dB) 2" <- w353
        "delta phase(deg) 2" <- w352
        n139 = TDMS Close(8:w362, 11:w363) -> (0:w359:errorcluster)  [unwired: 1 out]
      }
    }
    "state" <- w20
  }
  n140 = call <vilib>:"Simple Error Handler.vi"("error in (no error)"=w3) -> ()  [unwired: 4 in, 5 out]
